vi "Receive Value Change Event.vi"(8 "error in (no error)":errorcluster, 10 "ValueChangeMsg":refnum<class "ValueChangeMsg.lvclass">, 11 "MultiSubscriber In":refnum<class "MultiSubscriber.lvclass">) -> (0 "error out":errorcluster, 3 "MultiSubscriber Out":refnum<class "MultiSubscriber.lvclass">)   [LabVIEW 2018, in "TestViewables.lvlib" / "MultiSubscriber.lvclass"]
doc: "接收值更改事件"
uses:
  MultiSubscriber.lvclass
  modules/mva-viewable/Source/ActorEvents/IEventAggregator Messages/ValueChangeMsg/ValueChangeMsg.lvclass
  modules/mva-viewable/Source/ActorEvents/IEventAggregator Messages/ValueChangeMsg/ValueChangeMsg.lvclass/ValueChangeMsg.ctl
  modules/mva-viewable/Source/IViewable/IViewable/IViewable.lvclass
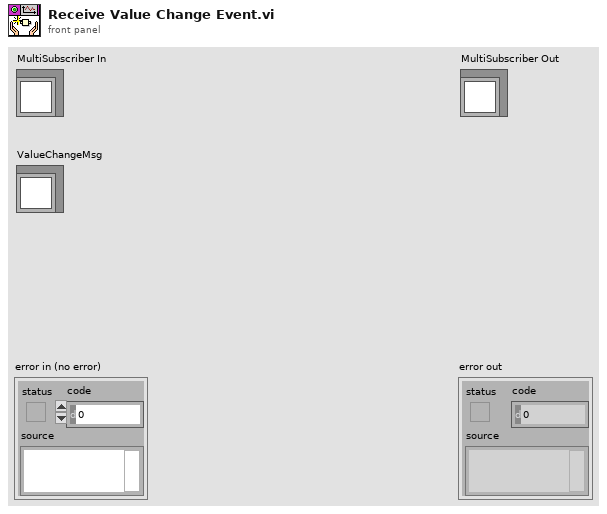
[diagram p1: front panel]
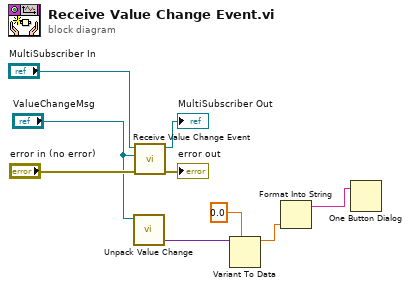
[diagram p0: block diagram]
diagram:
  n1 = call "Unpack Value Change.vi"("ValueChangeMsg"="ValueChangeMsg") -> ("New Value"=w4:variant)  [unwired: 6 in, 4 out]
  n2 = call-parent "Receive Value Change Event.vi"("error in (no error)"="error in (no error)", "ValueChangeMsg"="ValueChangeMsg", "IViewable In"="MultiSubscriber In") -> ("error out"=→"error out":errorcluster, "IViewable Out"=→"MultiSubscriber Out":refnum<class "MultiSubscriber.lvclass">)  [unwired: 7 in]
  n3 = Variant To Data(type=0.0, Variant=w4) -> (data=w2:dbl)  [unwired: 1 in, 1 out]
  n4 = Format Into String(w2) -> (resulting string=w1:string)  [unwired: 3 in, 1 out]
  n5 = One Button Dialog(message=w1) -> ()  [unwired: 1 in, 1 out]
